vi "Initialize.vi"(8 "error in (no error)":errorcluster, 9 "Timeout (2500ms)":i32=2500, 10 "Port (4223)":u16=4223, 11 "IP (localhost)":string="localhost") -> (0 "error out":errorcluster, 3 "IP Connection out":refnum<class "IP Connection.lvclass">)   [LabVIEW 2011, in "Tinkerforge.lvlib" / "IP Connection.lvclass"]
doc: "This VI initializes a <B>IP Connction</B> class object. It connects to the Brickd and calls the communication worker VI."
uses:
  IP Connection.lvclass
  IP Connection.lvclass/IP Connection.ctl
  Type Definitions/Errors.ctl
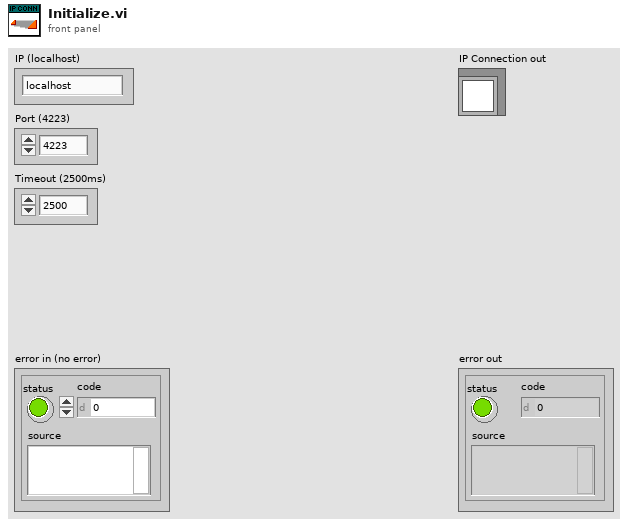
[diagram p1: front panel]
types:
  T1 = typedef "Tinkerforge.lvlib/IP Connection.lvclass/Errors.ctl" = enum16{"Timeout", "Device type incorrect", "Device already added", "Device not existing"}
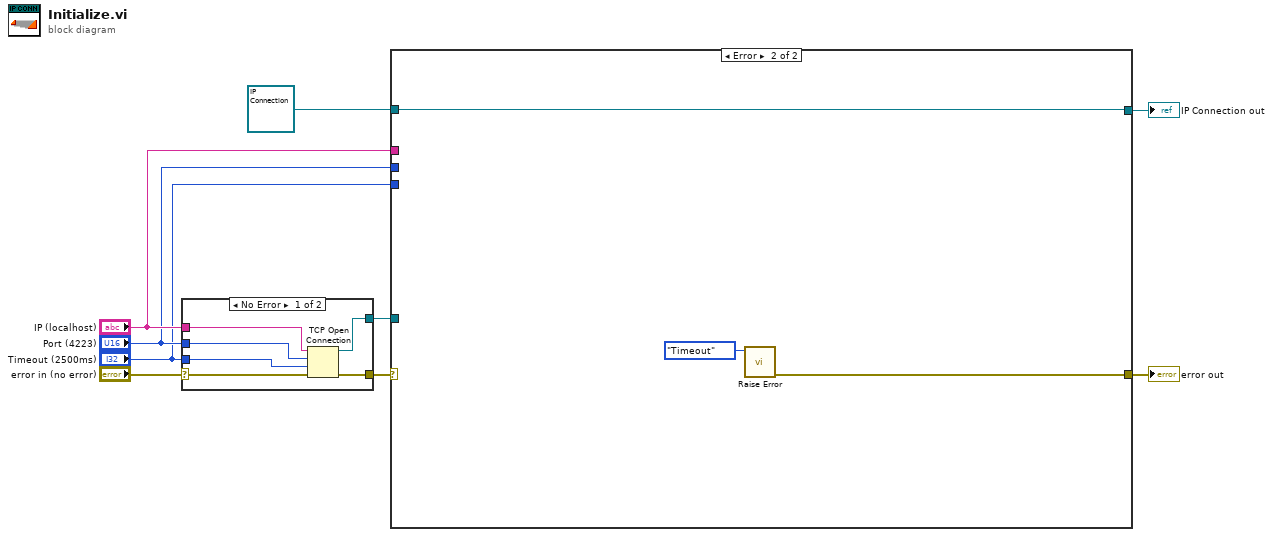
[diagram p0: block diagram]
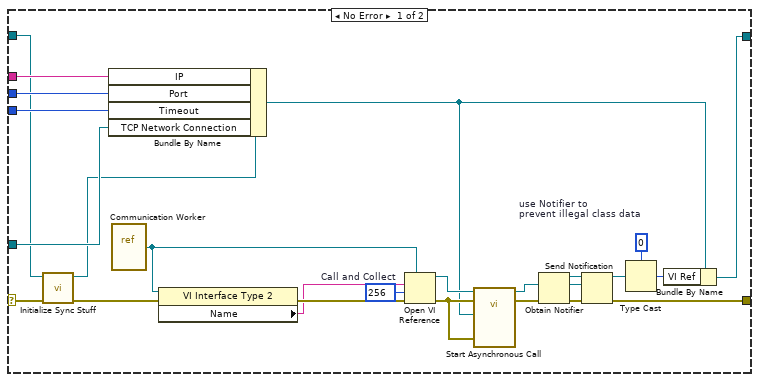
[diagram p2: hidden frame]
diagram:
  n1 = case shown="No Error" "error in (no error)" {
    selector: "error in (no error)" -> [w15 w16]
    tunnel: [w14 w16] -> w1
    tunnel: "IP (localhost)" -> [w13 _]
    tunnel: "Port (4223)" -> [w12 _]
    tunnel: "Timeout (2500ms)" -> [w11 _]
    tunnel: [w10 _] -> w4
    frame No Error {
      n2 = TCP Open Connection(address=w13, remote port or service name=w12, timeout ms (60000)=w11, error in (no error)=w15) -> (connection ID=w10:refnum<k5>, error out=w14:errorcluster)  [unwired: 1 in]
    }
    frame Error {
    }
  }
  n3 = case shown="Error" w1 {
    selector: w1 -> [w23 _]
    tunnel: [w18 w42] -> w8
    tunnel: "IP (localhost)" -> [w40 _]
    tunnel: "Port (4223)" -> [w39 _]
    tunnel: "Timeout (2500ms)" -> [w38 _]
    tunnel: refnum<class "IP Connection.lvclass"> refnum ("Tinkerforge.lvlib:IP Connection.lvclass") -> [w21 w43]
    tunnel: w4 -> [w37 _]
    tunnel: [w19 w43] -> w3
    frame No Error {
      w25 = u32 0  # use Notifier to prevent illegal class data
      w36 = 256  # Call and Collect
      n4 = call "Initialize Sync Stuff.vi"("error in (no error)"=w23, "IP Connection in"=w21) -> ("error out"=w22:errorcluster, "IP Connection out"=w20:refnum<class "IP Connection.lvclass">)  [unwired: 8 in]
      n5 = Bundle By Name(cluster=w20, "IP"=w40, "Port"=w39, "Timeout"=w38, "TCP Network Connection"=w37) -> (w30:refnum<class "IP Connection.lvclass">)
      n6 = vi-ref "Communication Worker.vi"() -> (w31:refnum<vi>)
      n7 = property class="VI Interface Type 2"(reference=w31, error in=w22) -> (error out=w33:errorcluster, "Name"=w32:string)  [unwired: 1 out]
      n8 = Open VI Reference(type specifier VI Refnum (for type only)=w31, vi path=w32, options=w36, error in (no error)=w33) -> (vi reference=w35:refnum<vi>, error out=w34:errorcluster)  [unwired: 2 in]
      n9 = call-by-ref "Start Asynchronous Call"(reference=w35, error in=w34, 8:"error in (no error)"=w34, "IP Connection in"=w30) -> (reference out=w17:refnum<vi>, error out=w29:errorcluster)  [unwired: 8 in, 2 out]
      n10 = Obtain Notifier(notification data type=w17, error in (no error)=w29) -> (notifier out=w27:refnum<notifier>, error out=w28:errorcluster)  [unwired: 2 in, 1 out]
      n11 = Send Notification(notification=w17, notifier=w27, error in (no error)=w28) -> (notifier out=w26:refnum<notifier>, error out=w18:errorcluster)
      n12 = Type Cast(type=w25, x=w26) -> (*(type *) &x=w24:u32)
      n13 = Bundle By Name(cluster=w30, "VI Ref"=w24) -> (w19:refnum<class "IP Connection.lvclass">)
    }
    frame Error {
      n14 = call "Raise Error.vi"("Error"=Errors."Timeout") -> ("Error Out"=w42:errorcluster)  [unwired: 10 in]
    }
  }
  "error out" <- w8
  "IP Connection out" <- w3
